vi "data_distributor_naive.vi"(8 "error in":errorcluster, 9 "Indicies":T3[](array[typedef]), 11 "Analog Data Array In":T6[](array[typedef])) -> (0 "error out":errorcluster, 1 "Pressure/Temperature/Mixture Properties":T2, 2 "Measurements Data":T1, 4 "Liquid Flow":cluster{"Average":dbl, "Average":dbl}, 5 "Diode Charts":T4, 6 "Vapor Flow":cluster{"Average":dbl, "Average":dbl}, 7 "Pulse Generator Charts":T5={"Vapor Mass Flow Rates"={"max value"=119484.80284900061, "max value"=11360.460004869077}, "Test Section Thermocouples"={"max value"=0.0, "max value"=0.0, "max value"=0.0}, "Pulse Generator Abs Pressure"=[], "Test Section Saturation Pressures"={"max value"=0.0, "max value"=0.0}})   [LabVIEW 2017]
uses:
  analog_data.ctl
  Utility Sub VIs/pulse_generator_data_charts.ctl
  Utility Sub VIs/diode_charts.ctl
  index_array_cluster.ctl
  Utility Sub VIs/pressure_temp_mixture.ctl
  Utility Sub VIs/pulse_generator_data.ctl
panel:
  # "Pulse Gen"
  # "Test Section"
  # "Saturation\nPressure [Pa]"
  # "Saturation\nTemperature [C]"
  # "Pressure [Pa]"
  # "Temperature [C]"
  # "Liquid Tank"
  # "Separator"
  # "Liquid Inlet"
  # "Vapor Tank"
  # "Vapor Inlet"
  # "Test Section"
  # "Upper Dev Section"
  # "Lower Dev Section"
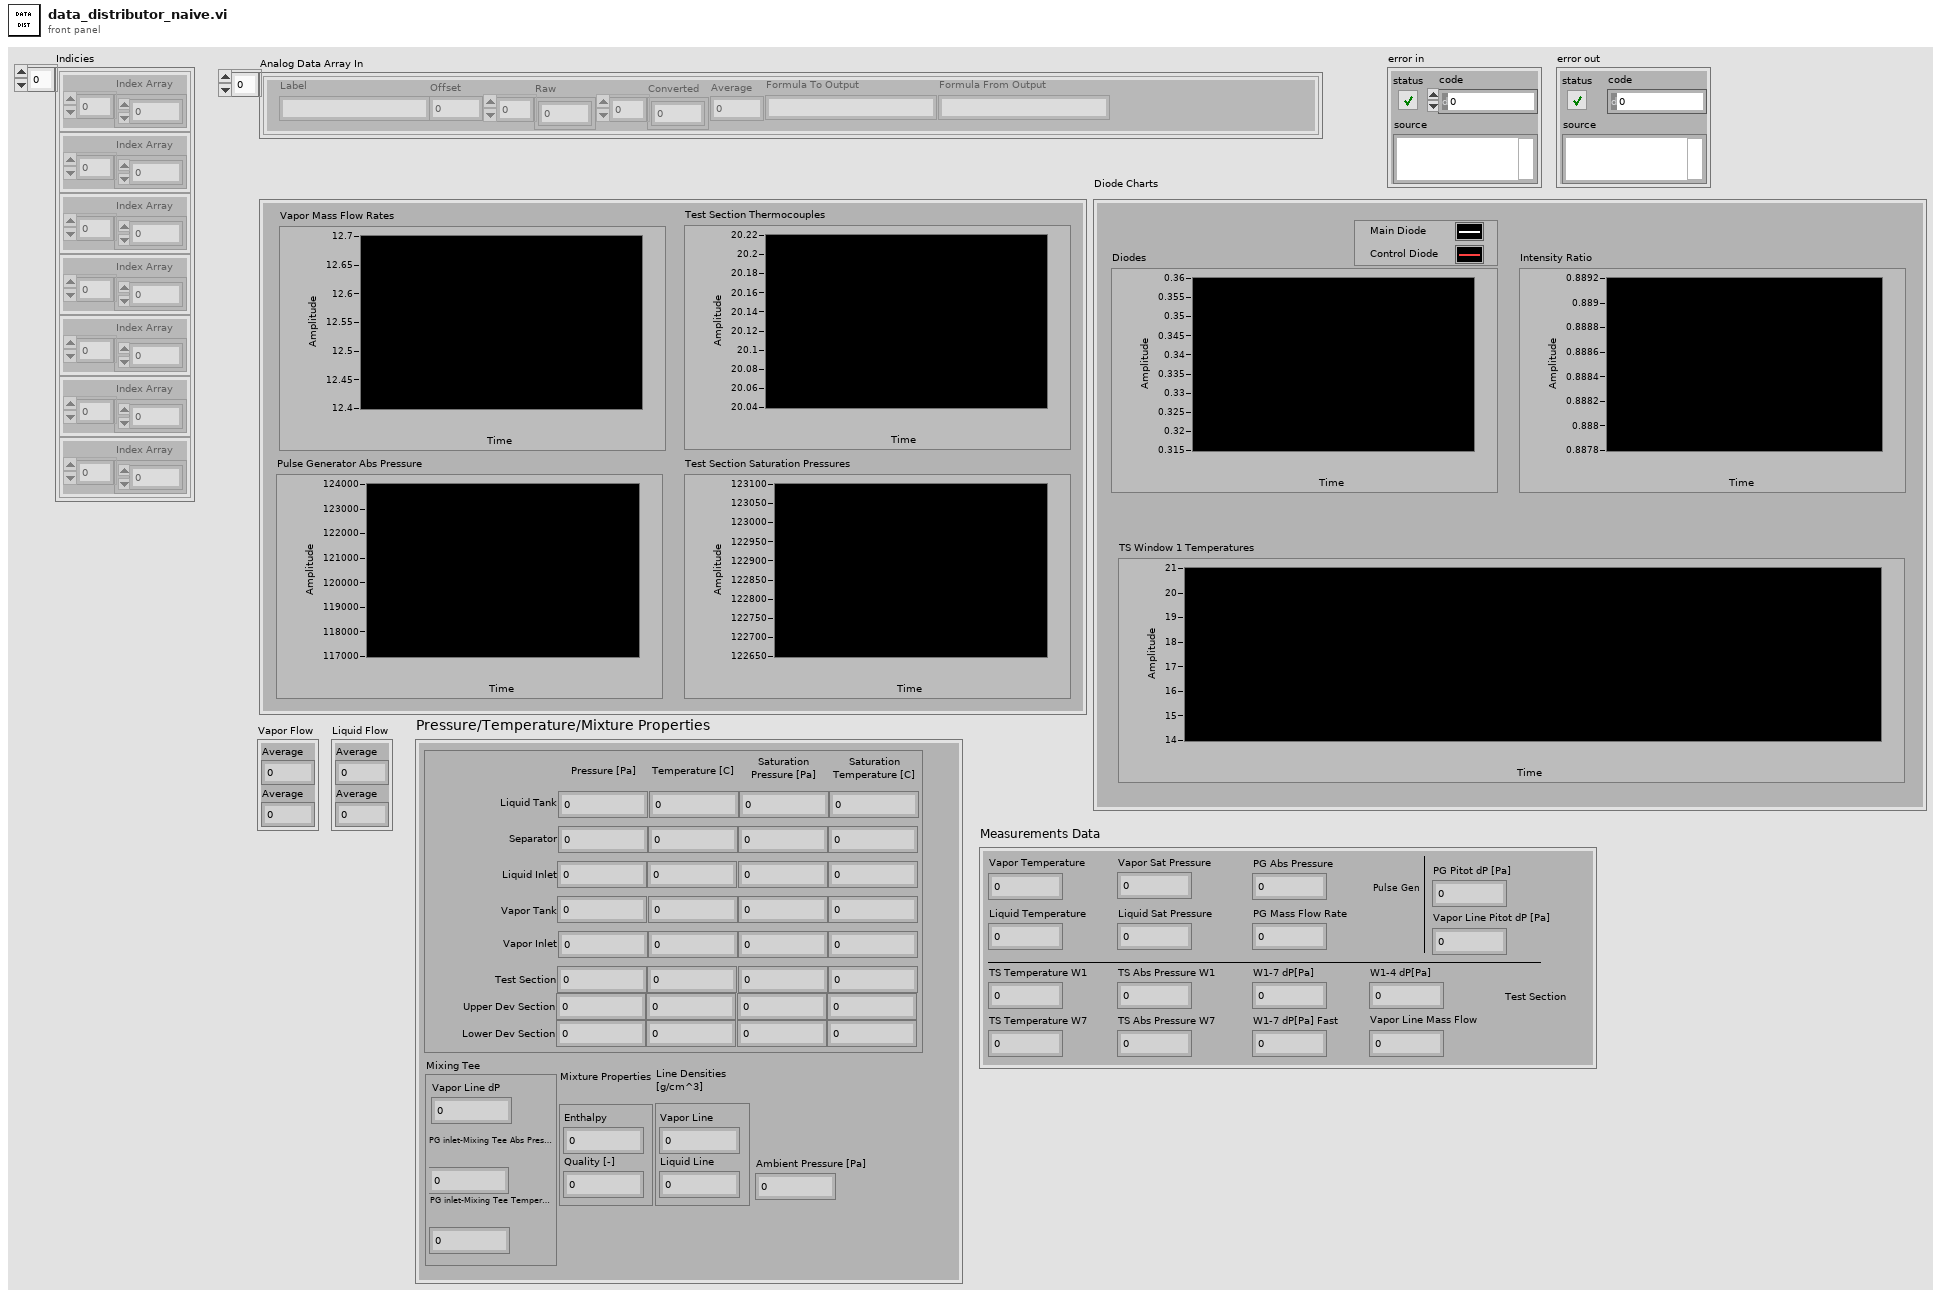
[diagram p1: front panel]
types:
  T1 = typedef "pulse_generator_data.ctl" = cluster{"PG Abs Pressure":dbl, "Vapor Temperature":dbl, "Liquid Temperature":dbl, "TS Temperature W1":dbl, "TS Temperature W7":dbl, "TS Abs Pressure W1":dbl, "TS Abs Pressure W7":dbl, "W1-4 dP[Pa]":dbl, "W1-7 dP[Pa]":dbl, "W1-7 dP[Pa] Fast":dbl, "PG Pitot dP [Pa]":dbl, "Vapor Line Pitot dP [Pa]":dbl, "Vapor Sat Pressure":dbl, "Liquid Sat Pressure":dbl, "PG Mass Flow Rate":dbl, "Vapor Line Mass Flow":dbl}
  T2 = typedef "pressure_temp_mixture.ctl" = cluster{"Line Densities\n[g/cm^3]":cluster{"Vapor Line":dbl, "Liquid Line":dbl}, "Mixture Properties":cluster{"Enthalpy":dbl, "Quality [-]":dbl}, "Component PTs":cluster{"Liquid Tank P":dbl, "Liquid Tank T":dbl, "Liquid Tank Sat P":dbl, "Liquid Tank Sat T":dbl, "Separator P":dbl, "Separator T":dbl, "Separator Sat P":dbl, "Separator Sat T":dbl, "Liquid Inlet P":dbl, "Liquid Inlet T":dbl, "Liquid Inlet Sat P":dbl, "Liquid Inlet Sat T":dbl, "Vapor Tank P":dbl, "Vapor Tank T":dbl, "Vapor Tank Sat P":dbl, "Vapor Tank Sat T":dbl, "Vapor Inlet P":dbl, "Vapor Inlet T":dbl, "Vapor Inlet Sat P":dbl, "Vapor Inlet Sat T":dbl, "Test Section P":dbl, "Test Section T":dbl, "Test Section Sat P":dbl, "Test Section Sat T":dbl, "Upper Dev Section P":dbl, "Upper Dev Section T":dbl, "Upper Dev Section Sat P":dbl, "Upper Dev Section Sat T":dbl, "Lower Dev Section P":dbl, "Lower Dev Section T":dbl, "Lower Dev Section Sat P":dbl, "Lower Dev Section Sat T":dbl}, "Ambient Pressure [Pa]":dbl, "Mixing Tee":cluster{"Vapor Line dP":dbl, "PG inlet-Mixing Tee Abs Pressure":dbl, "PG inlet-Mixing Tee Temperature":dbl}}
  T3 = typedef "index_array_cluster.ctl" = cluster{"Index Array":i32[]}
  T4 = typedef "diode_charts.ctl" = cluster{"Diodes":cluster{dbl, dbl}, "Intensity Ratio":dbl, "TS Window 1 Temperatures":cluster{"Average":dbl, "T Sat [C]":dbl}}
  T5 = typedef "pulse_generator_data_charts.ctl" = cluster{"Vapor Mass Flow Rates":cluster{"max value":dbl, "max value":dbl}, "Test Section Thermocouples":cluster{"max value":dbl, "max value":dbl, "max value":dbl}, "Pulse Generator Abs Pressure":dbl[], "Test Section Saturation Pressures":cluster{"max value":dbl, "max value":dbl}}
  T6 = typedef "analog_data.ctl" = cluster{"Label":string, "Offset":dbl, "Raw":dbl[], "Converted":dbl[], "Average":dbl, "Formula To Output":string, "Formula From Output":string}
  T7 = cluster{"Mixing Tee dP":dbl, "PG inlet-Mixing Tee Abs Pressure":dbl, "PG inlet-Mixing Tee Temperature":dbl}
  T8 = cluster{"[0]":dbl, "[1]":dbl, "[2]":dbl, "[3]":dbl, "[4]":dbl, "[5]":dbl, "[6]":dbl, "[7]":dbl, "[8]":dbl, "[9]":dbl, "[10]":dbl, "[11]":dbl, "[12]":dbl, "[13]":dbl, "[14]":dbl, "[15]":dbl, "[16]":dbl, "[17]":dbl, "[18]":dbl, "[19]":dbl, "[20]":dbl, "[21]":dbl, "[22]":dbl, "[23]":dbl, "[24]":dbl, "[25]":dbl, "[26]":dbl, "[27]":dbl, "[28]":dbl, "[29]":dbl, "[30]":dbl, "[31]":dbl}
  T9 = cluster{"Mass Flow Rate [g/s]":dbl, "Mass Flow Rate [g/s]":dbl}
  T10 = cluster{"[0]":dbl, "[1]":dbl, "[2]":dbl, "[3]":dbl, "[4]":dbl, "[5]":dbl, "[6]":dbl, "[7]":dbl, "[8]":dbl, "[9]":dbl, "[10]":dbl, "[11]":dbl, "[12]":dbl, "[13]":dbl, "[14]":dbl, "[15]":dbl}
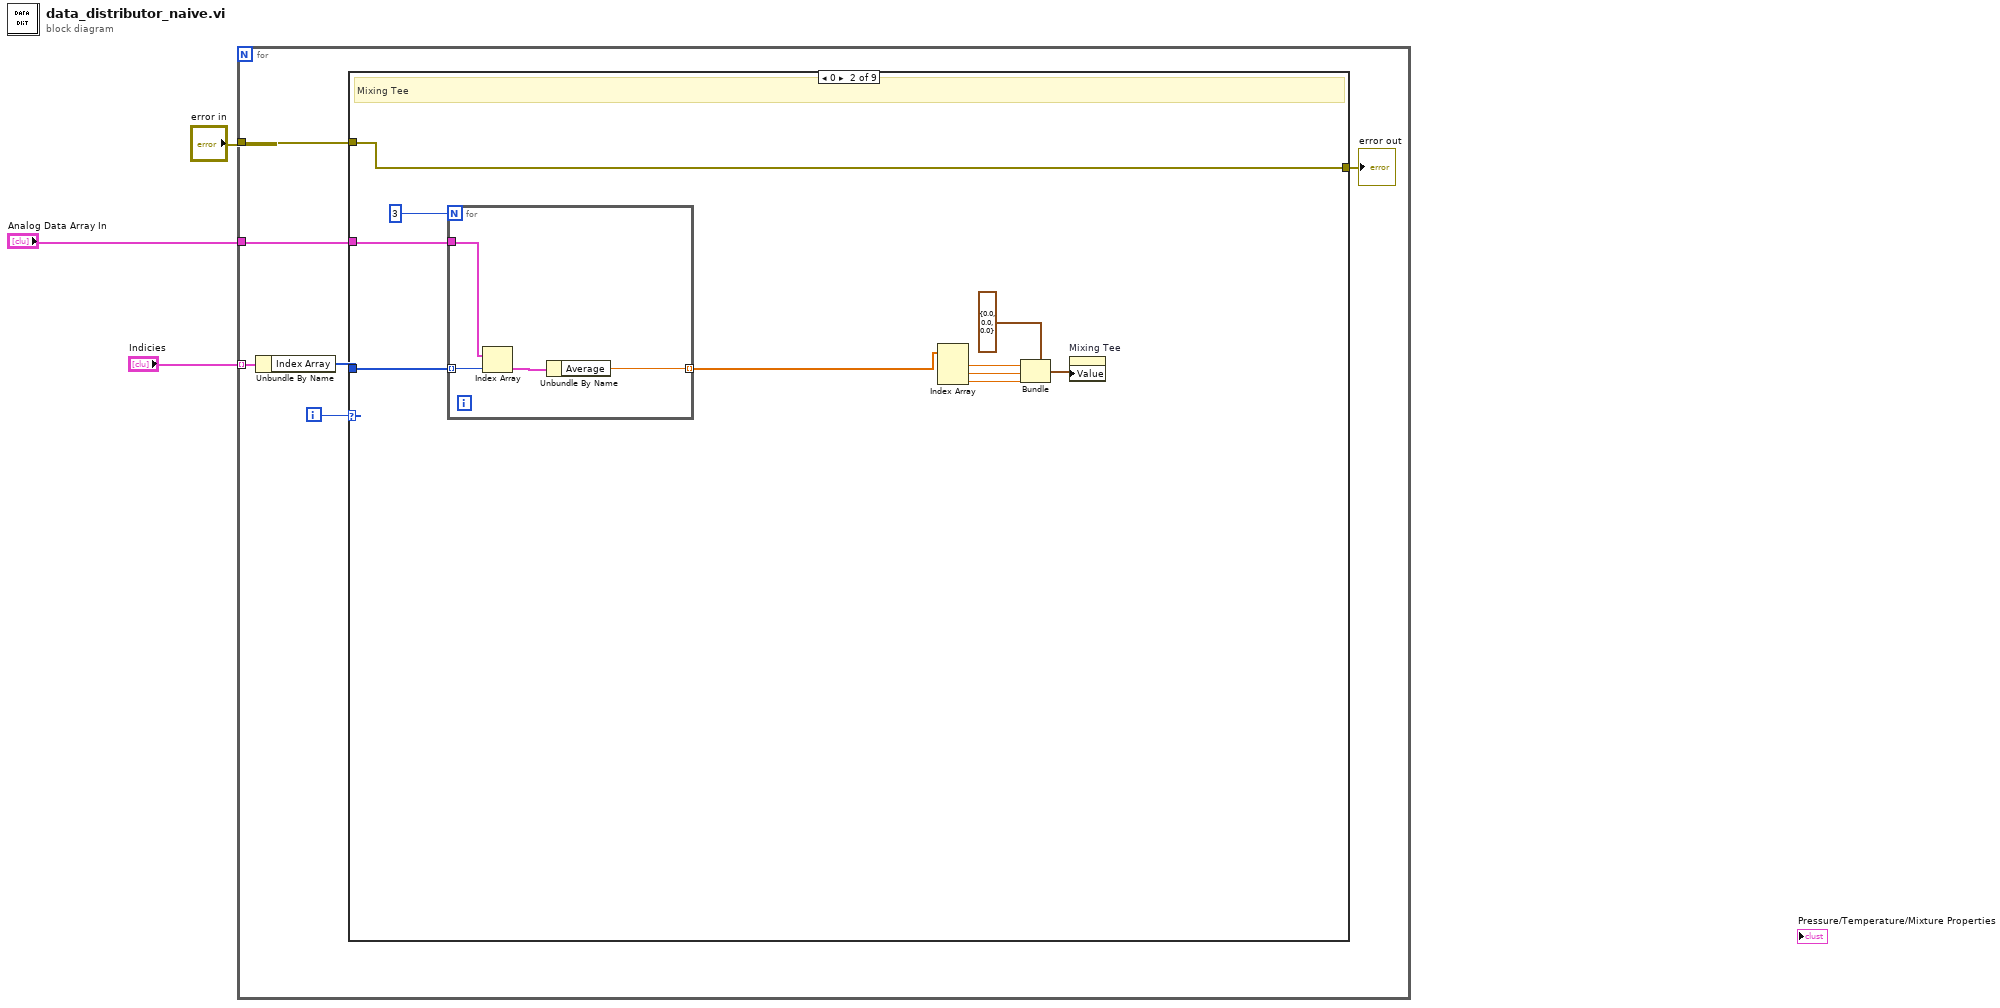
[diagram p0: block diagram]
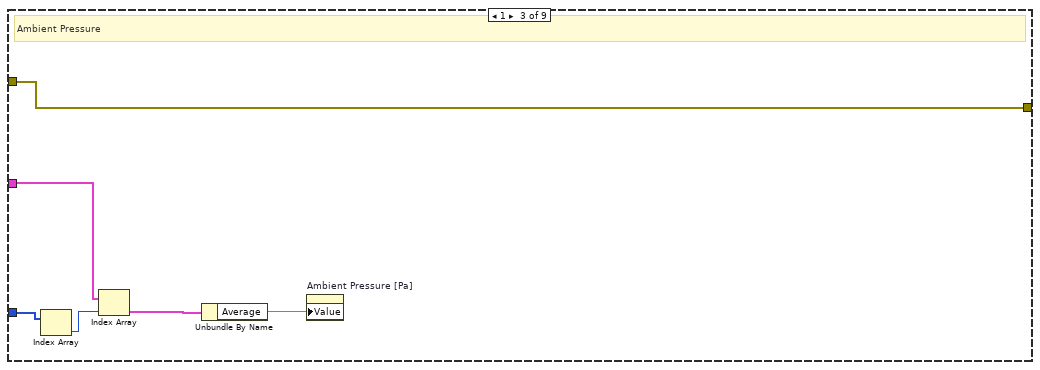
[diagram p3: hidden frame]
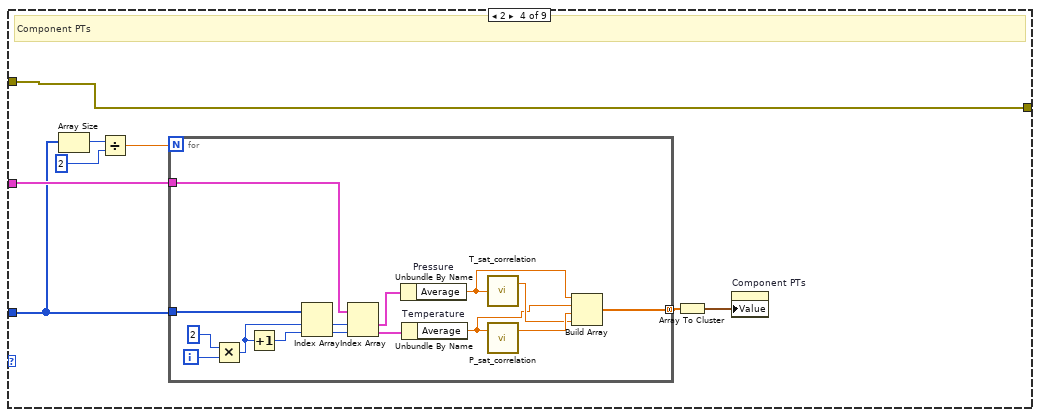
[diagram p4: hidden frame]
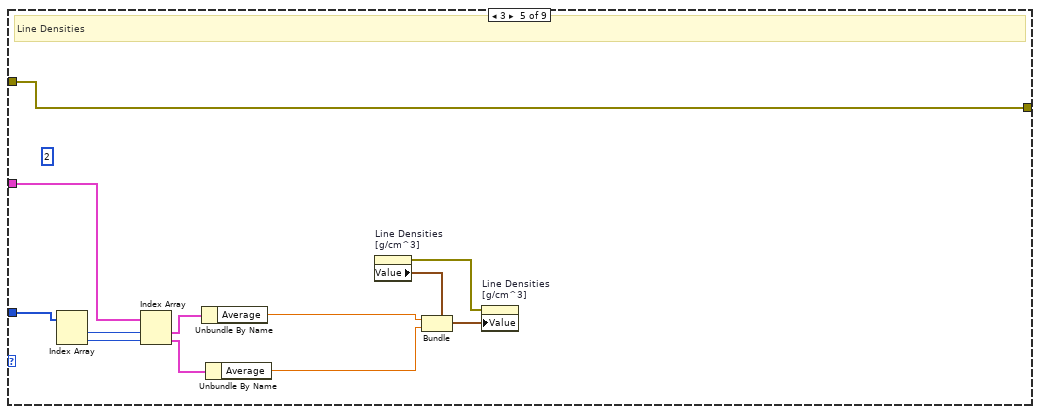
[diagram p5: hidden frame]
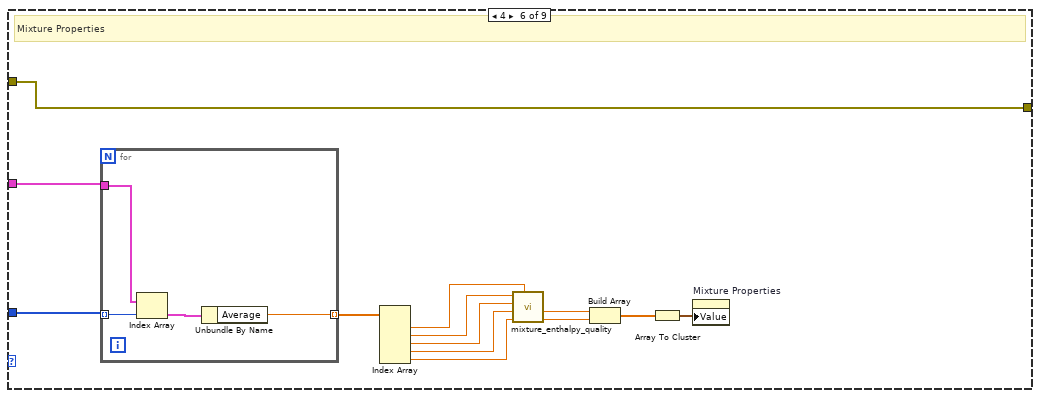
[diagram p6: hidden frame]
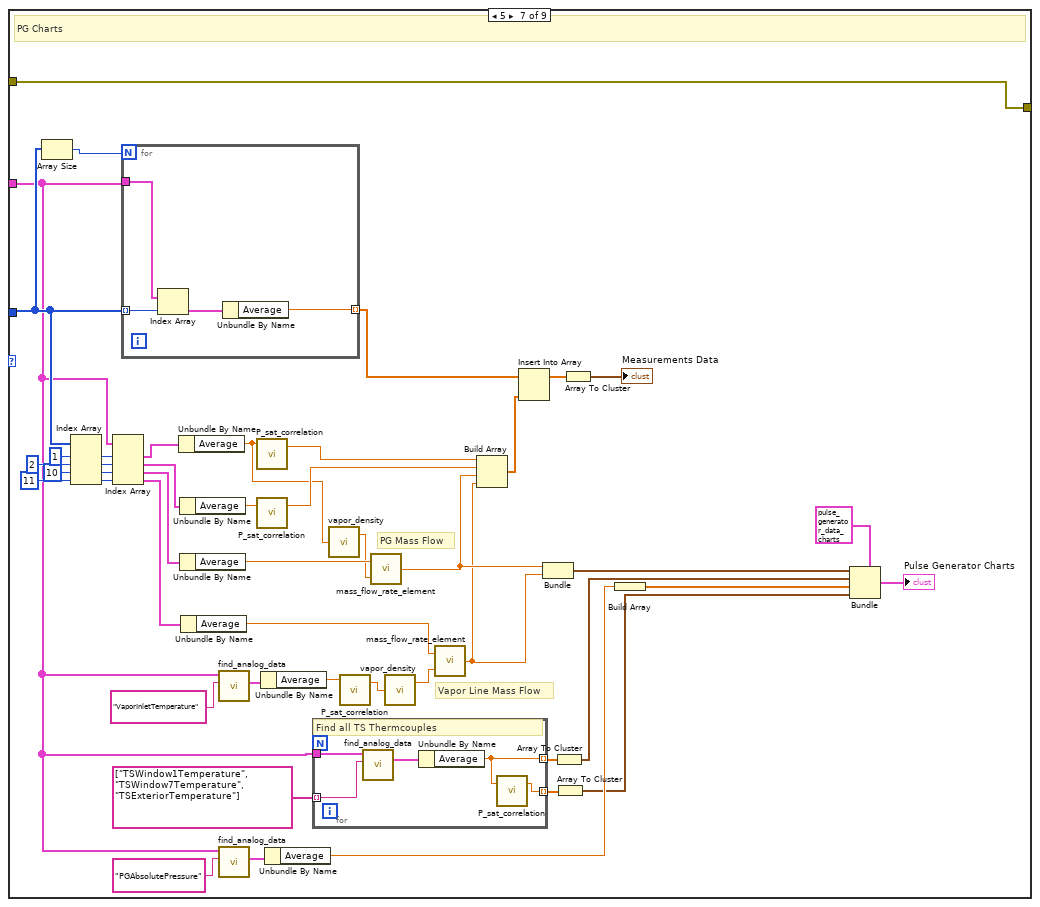
[diagram p7: hidden frame]
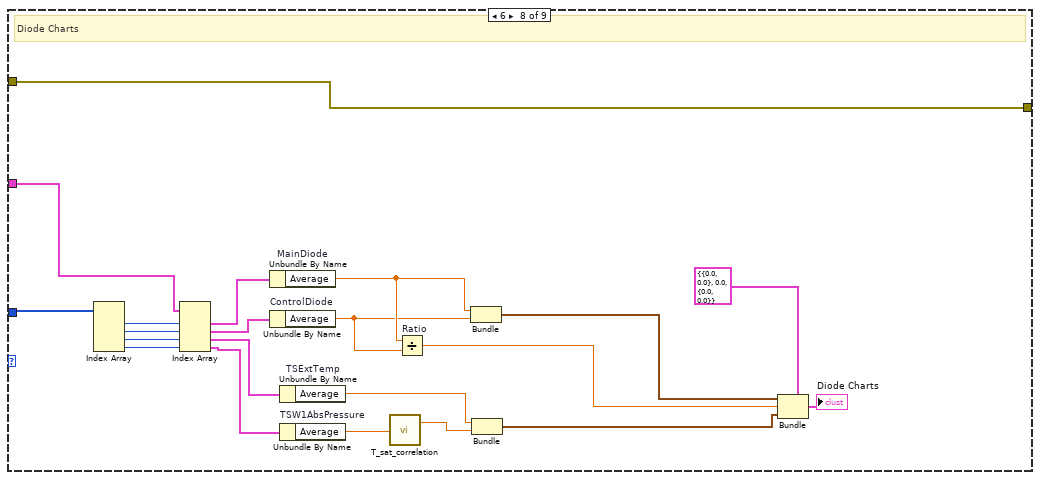
[diagram p8: hidden frame]
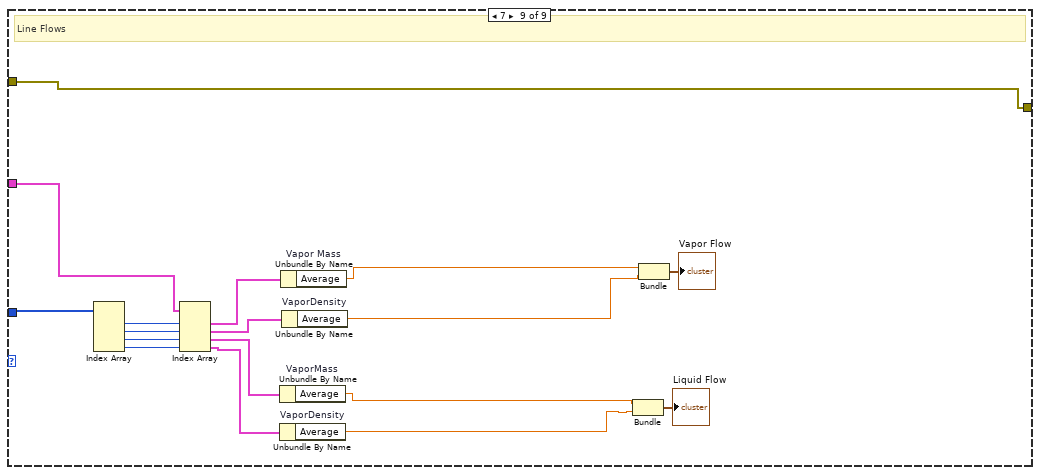
[diagram p9: hidden frame]
diagram:
  n1 = for {
    tunnel: "error in" -> [w9]
    tunnel: "Analog Data Array In" -> [w8]
    tunnel: "Indicies" -> [w5] mode=indexing
    i -> [w4]
    n2 = Unbundle By Name(w5) -> ("Index Array"=w6:i32[])
    n3 = case shown="0" w4 {
      tunnel: w6 -> [_ w20 w28 w37 w62 w77 w97 w158 w175]
      tunnel: w8 -> [_ w19 w30 w38 w59 w78 w87 w156 w173]
      tunnel: w9 -> [w10 w12 w26 w32 w63 w67 w98 w143 w161]
      tunnel: [w10 w12 w26 w32 w63 w67 w98 w143 w161] -> w7
      frame Default {
      }
      frame 0 {
        # "Mixing Tee"
        n4 = for {
          N: 3 -> [_]
          tunnel: w20 -> [w24] mode=indexing
          tunnel: w19 -> [w23]
          tunnel: [w21] -> w17 mode=indexing
          n5 = Index Array(array=w23, index=w24) -> (element=w22:T6)
          n6 = Unbundle By Name(w22) -> ("Average"=w21:dbl)
        }
        n7 = Index Array(array=w17) -> (element #1=w15:dbl, element #2=w14:dbl, element #3=w13:dbl)  [unwired: 3 in]
        n8 = Bundle(cluster=T7 {"Mixing Tee dP"=0.0, "PG inlet-Mixing Tee Abs Pressure"=0.0, "PG inlet-Mixing Tee Temperature"=0.0} ("Mixing Tee"), "Mixing Tee dP"=w15, "PG inlet-Mixing Tee Abs Pressure"=w14, "PG inlet-Mixing Tee Temperature"=w13) -> (w11:T7)
        n9 = property on="Mixing Tee" class="Clust (strict)"("Value"=w11) -> ()  [unwired: 2 in, 2 out]
      }
      frame 1 {
        # "Ambient Pressure"
        n10 = Index Array(array=w28) -> (element=w27:i32)  [unwired: 1 in]
        n11 = Index Array(array=w30, index=w27) -> (element=w29:T6)
        n12 = Unbundle By Name(w29) -> ("Average"=w25:dbl)
        n13 = property on="Ambient Pressure [Pa]" class="DigNum (strict)"("Value"=w25) -> ()  [unwired: 2 in, 2 out]
      }
      frame 2 {
        # "Component PTs"
        n14 = Array Size(array=w37) -> (size(s)=w35:i32)
        n15 = Divide(x=w35, y=2) -> (x/y=w36:dbl)
        n16 = for {
          N: w36 -> [_]
          tunnel: w37 -> [w49]
          tunnel: w38 -> [w53]
          tunnel: [w39] -> w33 mode=concatenating
          i -> [w51]
          n17 = Multiply(x=2, y=w51) -> (x*y=w47:i32)
          n18 = Increment(x=w47) -> (x+1=w48:i32)
          n19 = Index Array(array=w49, index #1=w47, index #2=w48) -> (element #1=w46:i32, element #2=w45:i32)
          n20 = Index Array(array=w53, index #1=w46, index #2=w45) -> (element #1=w52:T6, element #2=w44:T6)
          n21 = Unbundle By Name "Pressure"(w52) -> ("Average"=w41:dbl)
          n22 = Unbundle By Name "Temperature"(w44) -> ("Average"=w40:dbl)
          n23 = call "T_sat_correlation.vi"("P [Pa]"=w41) -> ("T Sat [C]"=w42:dbl)  [unwired: 1 out]
          n24 = call "P_sat_correlation.vi"("Temperature[C]"=w40) -> ("P Sat[Pa]"=w43:dbl)  [unwired: 1 in, 1 out]
          n25 = Build Array(w41, w40, w43, w42) -> (w39:dbl[])
        }
        n26 = Array To Cluster(array=w33) -> (cluster=w31:T8)
        n27 = property on="Component PTs" class="Clust (strict)"("Value"=w31) -> ()  [unwired: 2 in, 2 out]
      }
      frame 3 {
        (unwired) 2
        # "Line Densities"
        n28 = Index Array(array=w62) -> (element #1=w60:i32, element #2=w61:i32)  [unwired: 2 in]
        n29 = Index Array(array=w59, index #1=w60, index #2=w61) -> (element #1=w58:T6, element #2=w57:T6)
        n30 = Unbundle By Name(w58) -> ("Average"=w65:dbl)
        n31 = Unbundle By Name(w57) -> ("Average"=w64:dbl)
        n32 = property on="Line Densities\n[g/cm^3]" class="Clust (strict)"() -> (error out=w55:errorcluster, "Value"=w54:cluster{"Vapor Line":dbl, "Liquid Line":dbl})  [unwired: 2 in, 1 out]
        n33 = Bundle(cluster=w54, "Vapor Line"=w65, "Liquid Line"=w64) -> (w56:cluster{"Vapor Line":dbl, "Liquid Line":dbl})
        n34 = property on="Line Densities\n[g/cm^3]" class="Clust (strict)"(error in=w55, "Value"=w56) -> ()  [unwired: 1 in, 2 out]
      }
      frame 4 {
        # "Mixture Properties"
        n35 = for {
          tunnel: w77 -> [w82] mode=indexing
          tunnel: w78 -> [w81]
          tunnel: [w79] -> w76 mode=indexing
          n36 = Index Array(array=w81, index=w82) -> (element=w80:T6)
          n37 = Unbundle By Name(w80) -> ("Average"=w79:dbl)
        }
        n38 = Index Array(array=w76) -> (element #1=w72:dbl, element #2=w71:dbl, element #3=w70:dbl, element #4=w69:dbl, element #5=w68:dbl)  [unwired: 5 in]
        n39 = call "mixture_enthalpy_quality.vi"("Vapor Inlet Pressure [Pa]"=w72, "Separator Temp [C]"=w68, "Liquid Inlet Temp [C]"=w69, "Vapor Flow Rate [g/s]"=w70, "Liquid Flow Rate [g/s]"=w71) -> ("Quality [-]"=w74:dbl, "mixture enthalpy"=w75:dbl)  [unwired: 2 out]
        n40 = Build Array(w75, w74) -> (w73:dbl[])
        n41 = Array To Cluster(array=w73) -> (cluster=w66:cluster{"[0]":dbl, "[1]":dbl})
        n42 = property on="Mixture Properties" class="Clust (strict)"("Value"=w66) -> ()  [unwired: 2 in, 2 out]
      }
      frame 5 {
        # "Vapor Line Mass Flow"
        # "PG Mass Flow"
        # "PG Charts"
        n43 = Array Size(array=w97) -> (size(s)=w105:i32)
        n44 = Index Array(array=w97, index #1=1 ("index"), index #2=2 ("index"), index #3=10 ("index"), index #4=11 ("index")) -> (element #1=w96:i32, element #2=w91:i32, element #3=w90:i32, element #4=w89:i32)
        n45 = Index Array(array=w87, index #1=w96, index #2=w91, index #3=w90, index #4=w89) -> (element #1=w88:T6, element #2=w86:T6, element #3=w85:T6, element #4=w84:T6)
        n46 = for {
          N: w105 -> [_]
          tunnel: w97 -> [w137] mode=indexing
          tunnel: w87 -> [w136]
          tunnel: [w134] -> w119 mode=indexing
          n47 = Index Array(array=w136, index=w137) -> (element=w135:T6)
          n48 = Unbundle By Name(w135) -> ("Average"=w134:dbl)
        }
        n49 = Unbundle By Name(w88) -> ("Average"=w106:dbl)
        n50 = Unbundle By Name(w86) -> ("Average"=w128:dbl)
        n51 = Unbundle By Name(w85) -> ("Average"=w127:dbl)
        n52 = Unbundle By Name(w84) -> ("Average"=w120:dbl)
        n53 = call "find_analog_data.vi"("Needle"="VaporInletTemperature", "Haystack"=w87) -> ("Needle Out"=w124:T6)  [unwired: 7 in, 2 out]
        n54 = call "find_analog_data.vi"("Needle"="PGAbsolutePressure", "Haystack"=w87) -> ("Needle Out"=w113:T6)  [unwired: 7 in, 2 out]
        n55 = call "P_sat_correlation.vi"("Temperature[C]"=w106) -> ("P Sat[Pa]"=w118:dbl)  [unwired: 1 in, 1 out]
        n56 = call "P_sat_correlation.vi"("Temperature[C]"=w128) -> ("P Sat[Pa]"=w117:dbl)  [unwired: 1 in, 1 out]
        n57 = Unbundle By Name(w124) -> ("Average"=w123:dbl)
        n58 = Unbundle By Name(w113) -> ("Average"=w112:dbl)
        n59 = for {
          tunnel: string[] ["TSWindow1Temperature", "TSWindow7Temperature", "TSExteriorTemperature"] ("Needle") -> [w132] mode=indexing
          tunnel: w87 -> [w133]
          tunnel: [w130] -> w108 mode=indexing
          tunnel: [w129] -> w107 mode=indexing
          # "Find all TS Thermcouples"
          n60 = call "find_analog_data.vi"("Needle"=w132, "Haystack"=w133) -> ("Needle Out"=w131:T6)  [unwired: 7 in, 2 out]
          n61 = Unbundle By Name(w131) -> ("Average"=w130:dbl)
          n62 = call "P_sat_correlation.vi"("Temperature[C]"=w130) -> ("P Sat[Pa]"=w129:dbl)  [unwired: 1 in, 1 out]
        }
        n63 = call "vapor_density.vi"("Vapor Temp [C]"=w106) -> ("Vapor Density[g/cm3]"=w126:dbl)  [unwired: 1 out]
        n64 = call "P_sat_correlation.vi"("Temperature[C]"=w123) -> ("P Sat[Pa]"=w122:dbl)  [unwired: 1 in, 1 out]
        n65 = call "mass_flow_rate_element.vi"("Density [g/cm3]"=w126, "dP [Pa]"=w127) -> ("Mass Flow Rate [g/s]"=w111:dbl)
        n66 = call "vapor_density.vi"("Vapor Temp [C]"=w122) -> ("Vapor Density[g/cm3]"=w121:dbl)  [unwired: 1 out]
        n67 = call "mass_flow_rate_element.vi"("Density [g/cm3]"=w121, "dP [Pa]"=w120) -> ("Mass Flow Rate [g/s]"=w110:dbl)
        n68 = Build Array(w118, w117, w111, w110) -> (w116:dbl[])
        n69 = Insert Into Array(array=w119, new element=w116) -> (w115:dbl[])  [unwired: 1 in]
        n70 = Bundle("Mass Flow Rate [g/s]"=w111, "Mass Flow Rate [g/s]"=w110) -> (w102:T9)  [unwired: 1 in]
        n71 = Array To Cluster(array=w108) -> (cluster=w101:cluster{"[0]":dbl, "[1]":dbl, "[2]":dbl})
        n72 = Array To Cluster(array=w107) -> (cluster=w99:cluster{"[0]":dbl, "[1]":dbl})
        n73 = Array To Cluster(array=w115) -> (cluster=→"Measurements Data":T10)
        n74 = Build Array(w112) -> (w100:dbl[])
        n75 = Bundle(cluster=T5 {"Vapor Mass Flow Rates"={"max value"=119484.80284900061, "max value"=11360.460004869077}, "Test Section Thermocouples"={"max value"=0.0, "max value"=0.0, "max value"=0.0}, "Pulse Generator Abs Pressure"=[], "Test Section Saturation Pressures"={"max value"=0.0, "max value"=0.0}} ("Pulse Generator Charts 2"), "Vapor Mass Flow Rates"=w102, "Test Section Thermocouples"=w101, "Pulse Generator Abs Pressure"=w100, "Test Section Saturation Pressures"=w99) -> (→"Pulse Generator Charts":T5)
      }
      frame 6 {
        # "Diode Charts"
        n76 = Index Array(array=w158) -> (element #1=w153:i32, element #2=w157:i32, element #3=w155:i32, element #4=w154:i32)  [unwired: 4 in]
        n77 = Index Array(array=w156, index #1=w153, index #2=w157, index #3=w155, index #4=w154) -> (element #1=w152:T6, element #2=w151:T6, element #3=w148:T6, element #4=w147:T6)
        n78 = Unbundle By Name "MainDiode"(w152) -> ("Average"=w150:dbl)
        n79 = Unbundle By Name "ControlDiode"(w151) -> ("Average"=w149:dbl)
        n80 = Unbundle By Name "TSExtTemp"(w148) -> ("Average"=w145:dbl)
        n81 = Unbundle By Name "TSW1AbsPressure"(w147) -> ("Average"=w146:dbl)
        n82 = call "T_sat_correlation.vi"("P [Pa]"=w146) -> ("T Sat [C]"=w144:dbl)  [unwired: 1 out]
        n83 = Divide "Ratio"(x=w150, y=w149) -> (x/y=w139:dbl)
        n84 = Bundle("Average"=w150, "Average"=w149) -> (w140:cluster{"Average":dbl, "Average":dbl})  [unwired: 1 in]
        n85 = Bundle("Average"=w145, "T Sat [C]"=w144) -> (w138:cluster{"Average":dbl, "T Sat [C]":dbl})  [unwired: 1 in]
        n86 = Bundle(cluster=T4 {"Diodes"={0.0, 0.0}, "Intensity Ratio"=0.0, "TS Window 1 Temperatures"={"Average"=0.0, "T Sat [C]"=0.0}} ("Diode Charts"), "Diodes"=w140, "Intensity Ratio"=w139, "TS Window 1 Temperatures"=w138) -> (→"Diode Charts":T4)
      }
      frame 7 {
        # "Line Flows"
        n87 = Index Array(array=w175) -> (element #1=w170:i32, element #2=w174:i32, element #3=w172:i32, element #4=w171:i32)  [unwired: 4 in]
        n88 = Index Array(array=w173, index #1=w170, index #2=w174, index #3=w172, index #4=w171) -> (element #1=w169:T6, element #2=w168:T6, element #3=w167:T6, element #4=w166:T6)
        n89 = Unbundle By Name "VaporMass"(w167) -> ("Average"=w163:dbl)
        n90 = Unbundle By Name "VaporDensity"(w166) -> ("Average"=w162:dbl)
        n91 = Unbundle By Name "Vapor Mass"(w169) -> ("Average"=w165:dbl)
        n92 = Unbundle By Name "VaporDensity"(w168) -> ("Average"=w164:dbl)
        n93 = Bundle("Average"=w163, "Average"=w162) -> (→"Liquid Flow":cluster{"Average":dbl, "Average":dbl})  [unwired: 1 in]
        n94 = Bundle("Average"=w165, "Average"=w164) -> (→"Vapor Flow":cluster{"Average":dbl, "Average":dbl})  [unwired: 1 in]
      }
    }
    "error out" <- w7
  }
